vi "getFileName.vi"(10 "File not found?":bool=TRUE, 11 "Path":path) -> (1 "NameTagFound":bool, 2 "SuccessfulRead?":bool, 3 "Filename":string)   [LabVIEW 2016]
uses:
  <vilib>/NI/GXML/_subVIs/GXML SearchParser/Search Parser.vi
  <vilib>/NI/GXML/GXML.lvlib
panel:
  # "Reads the name key from an XML file fetched from the target, which\ncontains the name of the file. Returns a warning if no file is found'or it does not\ncontain the element"
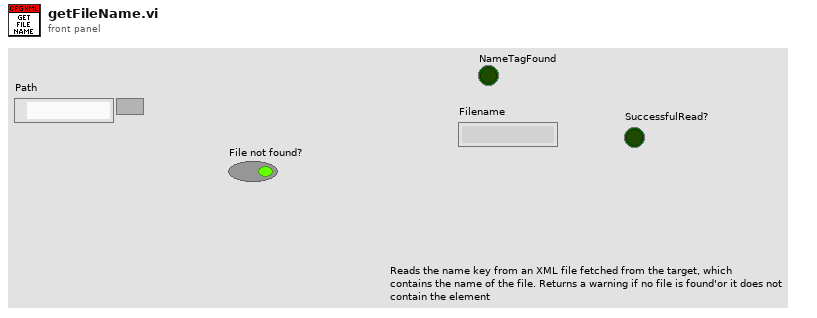
[diagram p1: front panel]
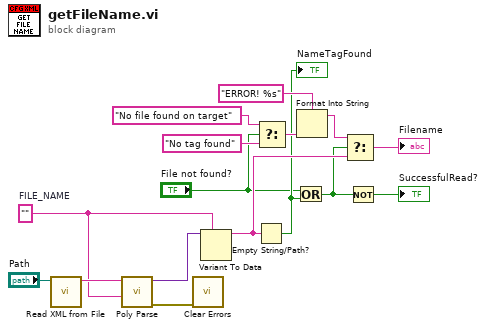
[diagram p0: block diagram]
diagram:
  w13 = ""  # FILE_NAME
  n1 = call <vilib>:"Read XML from File.vi"("XML File Path"="Path") -> ("XML String Out"=w15:string)  [unwired: 9 in, 1 out]
  n2 = call-poly <vilib>:"Poly Parse.vi"("TypeDesc"=w13, "XML String In"=w15) -> ("error out"=w4:errorcluster, "Parsed Data"=w14:variant)  [unwired: 8 in]
  n3 = call <vilib>:"Clear Errors.vi"("error in (no error)"=w4) -> ()  [unwired: 5 in, 2 out]
  n4 = Variant To Data(type=w13, Variant=w14) -> (data=w12:string)  [unwired: 1 in, 1 out]
  n5 = Empty String/Path?(string/path=w12) -> (empty?=w5:bool)
  "NameTagFound" <- w5
  n6 = Select(t="No file found on target", s="File not found?", f="No tag found") -> (s? t:f=w8:string)
  n7 = Or(x="File not found?", y=w5) -> (x .or. y?=w3:bool)
  n8 = Format Into String(format string="ERROR! %s", w8) -> (resulting string=w7:string)  [unwired: 2 in, 1 out]
  n9 = Select(t=w7, s=w3, f=w12) -> (s? t:f=→"Filename":string)
  n10 = Not(x=w3) -> (.not. x?=→"SuccessfulRead?":bool)
